vi "Enqueue Message.vi"   [LabVIEW 2014, in "MyQH Message Queue.lvlib"]
doc: "Normale Nachrichten werden an die Queue angehängt. Nachrichten mit hoher Priorität werden an den Anfang der Queue eingefügt."
uses:
  MyQH Message Queue.lvlib
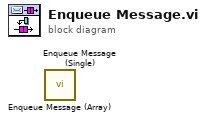
[diagram p0: block diagram]
diagram:
  n1 = call "Enqueue Message (Array).vi"() -> ()  [unwired: 10 in, 2 out]
  n2 = call "Enqueue Message (Single).vi"() -> ()  [unwired: 10 in, 2 out]
